vi "dashboard data.vi"() -> ()   [LabVIEW 2014]
panel:
  in  "Autonomous Mode":T1(ring)
  in  "Use Prog Laptop for Test":bool
  in  "Center Motor Output":dbl
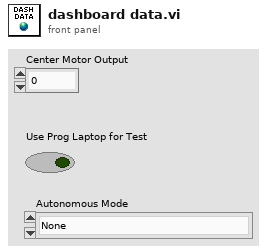
[diagram p1: front panel]
types:
  T1 = enum32{"None", "Autonomous 1 (Drive)", "Autonomous 2 (3 Tote)", "Autonomous 3 (Container)"}
diagram:
